vi "VCS Set Ipm Buffer Parameter.vi"(8 "error in (no error)":errorcluster, 10 "IPM buffer parameter":T1, 11 "axis in":cluster{"keyHandle":u32, "nodeId":u16}={"keyHandle"=0, "nodeId"=1}) -> (0 "error out":errorcluster, 3 "axis out":cluster{"keyHandle":u32, "nodeId":u16}={"keyHandle"=0, "nodeId"=1})   [LabVIEW 2019, in "maxonEPOS.lvlib"]
doc: "The function <B>VCS_SetIpmBufferParameter</B> sets warning borders of the data input."
uses:
  Examples/maxonEPOS.lvlib
  Resources/EposCmd.dll
  Resources/EposCmd64.dll
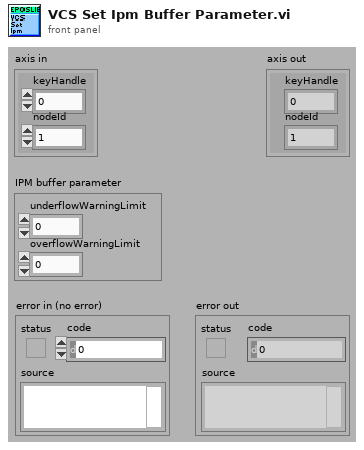
[diagram p1: front panel]
types:
  T1 = cluster{"underflowWarningLimit":u16, "overflowWarningLimit":u16}
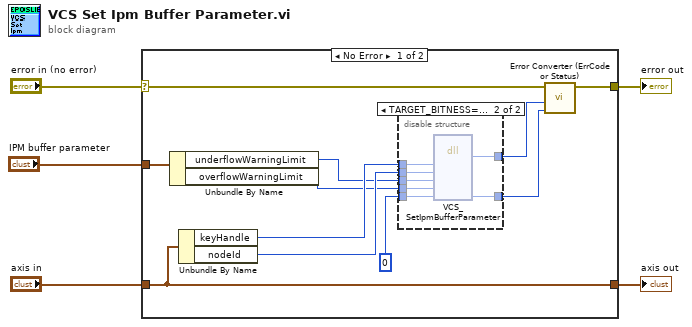
[diagram p0: block diagram]
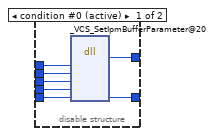
[diagram p2: hidden frame]
diagram:
  n1 = case shown="No Error" "error in (no error)" {
    selector: "error in (no error)" -> [w14 w31]
    tunnel: "axis in" -> [w16 w32]
    tunnel: [w16 w32] -> w4
    tunnel: [w15 w31] -> w3
    tunnel: "IPM buffer parameter" -> [w8 _]
    frame No Error {
      n2 = Unbundle By Name(w8) -> ("underflowWarningLimit"=w7:u16, "overflowWarningLimit"=w6:u16)
      n3 = Unbundle By Name(w16) -> ("keyHandle"=w11:u32, "nodeId"=w12:u16)
      n4 = disable-structure shown="TARGET_BITNESS==64" {
        disable-tunnel: u32 0 ("pErrorCode") -> [w23 w30]
        disable-tunnel: w12 -> [w22 w29]
        disable-tunnel: w11 -> [w21 w28]
        disable-tunnel: [w20 w27] -> w10
        disable-tunnel: [w19 w26] -> w9
        disable-tunnel: w7 -> [w18 w25]
        disable-tunnel: w6 -> [w17 w24]
        frame condition #0 (active) {
          n5 = dll-call lib="C:/workspace/project/scancon/sw/SSI_Tool/InstrumentsInterfaces/Motordriver/maxon EPOS/Resources/EposCmd.*" fn="_VCS_SetIpmBufferParameter@20"("KeyHandle"=w21, "NodeId"=w22, "UnderflowWarningLimit"=w18, "OverflowWarningLimit"=w17, "pErrorCode"=w23) -> (w20:i32, "pErrorCode"=w19:u32)  [unwired: 7 in, 2 out]
        }
        frame condition #1 {
          n6 = dll-call lib="C:/Sources/LabView/maxon EPOS/Resources/EposCmd64.*" fn="VCS_SetIpmBufferParameter" ("EposCmd.dll:_VCS_SetIpmBufferParameter@20")("KeyHandle"=w28, "NodeId"=w29, "UnderflowWarningLimit"=w25, "OverflowWarningLimit"=w24, "pErrorCode"=w30) -> ("Rückgabetyp"=w27:i32, "pErrorCode"=w26:u32)  [unwired: 7 in, 2 out]
        }
      }
      n7 = call "Error Converter (ErrCode or Status).vi"("error code"=w9, "return type"=w10, "error in (no error)"=w14) -> ("error out"=w15:errorcluster)  [unwired: 7 in]
    }
    frame Error {
    }
  }
  "error out" <- w3
  "axis out" <- w4
